vi "SP Get All Plots to Update.vi"(1 "Current Plot":refnum<vi>, 3 "Plot References":refnum<vi>[](array[refnum])) -> (0 "Plots to Update":refnum<vi>[](array[refnum]))   [LabVIEW 2011]
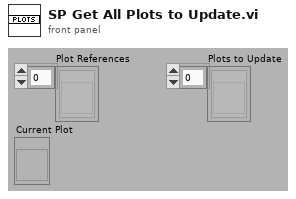
[diagram p1: front panel]
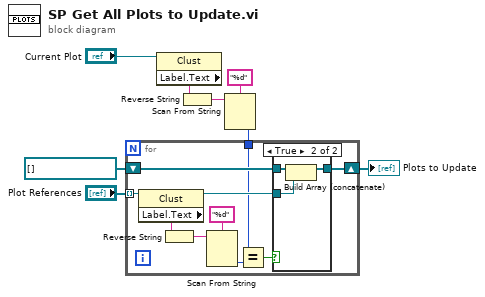
[diagram p0: block diagram]
diagram:
  n1 = property class="Clust"(reference="Current Plot") -> ("Label.Text"=w2:string)  [unwired: 1 in, 2 out]
  n2 = Reverse String(1:w2) -> (0:w3:string)
  n3 = Scan From String(format string="%d", input string=w3) -> (output 1=w1:i32)  [unwired: 2 in, 4 out]
  n4 = for {
    shift-right: [w17] -> w8
    shift-left: refnum<vi>[] [] -> [w18]
    tunnel: "Plot References" -> [w13] mode=indexing
    tunnel: w1 -> [w10]
    n5 = property class="Clust"(reference=w13) -> (reference out=w12:refnum<vi>, "Label.Text"=w16:string)  [unwired: 1 in, 1 out]
    n6 = Reverse String(1:w16) -> (0:w15:string)
    n7 = Scan From String(format string="%d", input string=w15) -> (output 1=w11:i32)  [unwired: 2 in, 4 out]
    n8 = Equal?(x=w10, y=w11) -> (x = y?=w9:bool)
    n9 = case shown="True" w9 {
      tunnel: w18 -> [w19 w22]
      tunnel: [w19 w21] -> w17
      tunnel: w12 -> [_ w20]
      frame False {
      }
      frame True {
        n10 = Build Array (concatenate)(w22, w20) -> (w21:refnum<vi>[])
      }
    }
  }
  "Plots to Update" <- w8
